vi "SaveFileDialogue.vi"(9 "文件参数":T1, 10 "文件路径":path, 11 "VI输入":refnum<vi>) -> (0 "错误输出":errorcluster, 2 "取消":bool, 3 "输出路径":path)   [LabVIEW 2020, in "Curve Editor.lvlib"]
uses:
  Curve Editor.lvlib
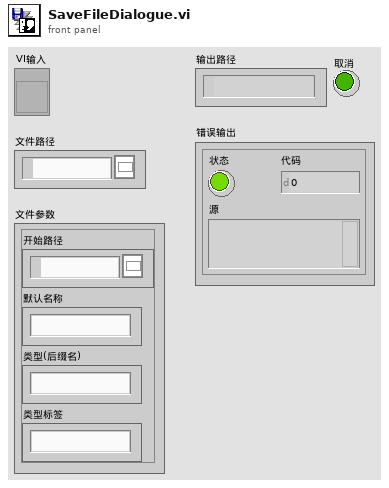
[diagram p1: front panel]
types:
  T1 = cluster{"开始路径":path, "默认名称":string, "类型(后缀名)":string, "类型标签":string}
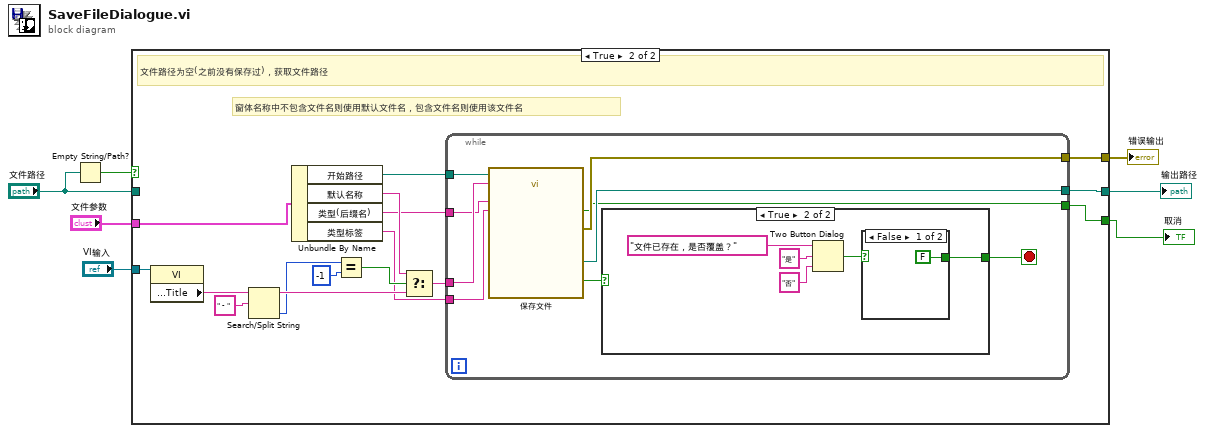
[diagram p0: block diagram]
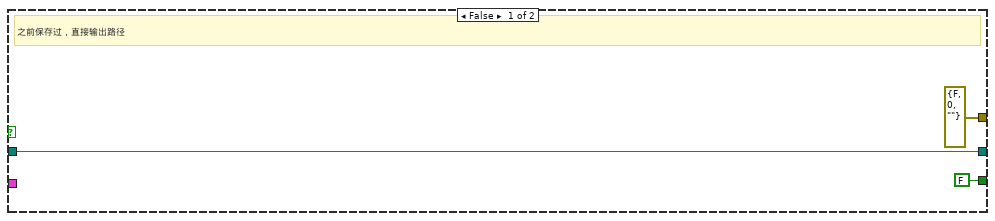
[diagram p2: hidden frame]
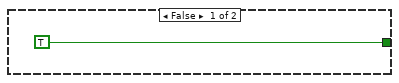
[diagram p3: hidden frame]
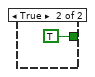
[diagram p4: hidden frame]
diagram:
  n1 = Empty String/Path?(string/path="文件路径") -> (empty?=w2:bool)
  n2 = case shown="True" w2 {
    tunnel: [w10 w13] -> w5
    tunnel: "文件路径" -> [w10 _]
    tunnel: [errorcluster {"status"=FALSE, "code"=0, "source"=""} ("error out") w12] -> w4
    tunnel: "VI输入" -> [_ w19]
    tunnel: "文件参数" -> [_ w18]
    tunnel: [FALSE ("cancelled") w11] -> w1
    frame False {
      # "之前保存过，直接输出路径"
    }
    frame True {
      # "窗体名称中不包含文件名则使用默认文件名，包含文件名则使用该文件名"
      # "文件路径为空(之前没有保存过)，获取文件路径"
      n3 = property class="VI"(reference=w19) -> ("Front Panel.Title"=w26:string)  [unwired: 1 in, 2 out]
      n4 = Search/Split String(string=w26, search string/char (-)=" - " ("搜索字符串/字符(-)")) -> (substring before match=w24:string, offset of match=w23:i32)  [unwired: 1 in, 1 out]
      n5 = Unbundle By Name(w18) -> ("开始路径"=w17:path, "默认名称"=w20:string, "类型(后缀名)"=w15:string, "类型标签"=w14:string)
      n6 = Equal?(x=w23, y=-1) -> (x = y?=w21:bool)
      n7 = Select(t=w20, s=w21, f=w24) -> (s? t:f=w16:string)
      n8 = while {
        tunnel: [w33] -> w12
        tunnel: [w32] -> w13
        tunnel: w17 -> [w31]
        tunnel: w16 -> [w30]
        tunnel: w15 -> [w29]
        tunnel: w14 -> [w28]
        tunnel: [w27] -> w11
        stop <- w35 stop-if-true
        n9 = call "保存文件"("start path"=w31, "default name"=w30, "pattern (all files)"=w29, "pattern label"=w28) -> ("selected path"=w32:path, "exists"=w34:bool, "cancelled"=w27:bool, "error out"=w33:errorcluster)  [unwired: 8 in]
        n10 = case shown="True" w34 {
          tunnel: [TRUE w37] -> w35
          frame False {
          }
          frame True {
            n11 = Two Button Dialog(message="文件已存在，是否覆盖？" ("消息"), 1:"否" ("F按钮名称（“取消”）"), 2:"是" ("T按钮名称（“确定”）")) -> (T button?=w38:bool)
            n12 = case shown="False" w38 {
              tunnel: [FALSE TRUE] -> w37
              frame False {
              }
              frame True {
              }
            }
          }
        }
      }
    }
  }
  "输出路径" <- w5
  "错误输出" <- w4
  "取消" <- w1
